vi "Type Conversion.From Double (1D Boolean).vi"(3 "values in":dbl[](array[numeric])) -> (1 "values out":bool[](array[boolean]))   [LabVIEW 2016, in "VeriStand Data.lvlib"]
doc: "Converts the provided double float values to the specified data type, preserving the numerical value of the data."
uses:
  VeriStand Data.lvlib
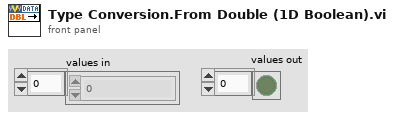
[diagram p1: front panel]
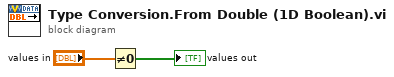
[diagram p0: block diagram]
diagram:
  n1 = Not Equal To 0?(x="values in") -> (x != 0?=→"values out":bool[])
